vi "16 - Fonts (Render As Texture).vi"() -> ()   [LabVIEW 2015]
uses:
  Libraries/LibSDL2 Wrapper/Controls/Rectangle.ctl
  Libraries/LibSDL2 Wrapper/Controls/Init Flags.ctl
  Libraries/LibSDL2 Wrapper/Controls/NULL.ctl
  Libraries/LibSDL2 Wrapper/LibSDL2.lvlib
  Libraries/LibSDL2_Image Wrapper/LibSDL2_Image.lvlib
  Libraries/LibSDL2_TTF Wrapper/LibSDL2_TTF.lvlib
panel:
  out "Period":dbl format="%.2p"
  in  "milliseconds to wait":u32=250
  in  "Destination Rectangle":T1
  in  "Colour":u32(colorbox)=16448250
  in  "stop":bool
  out "Error":string
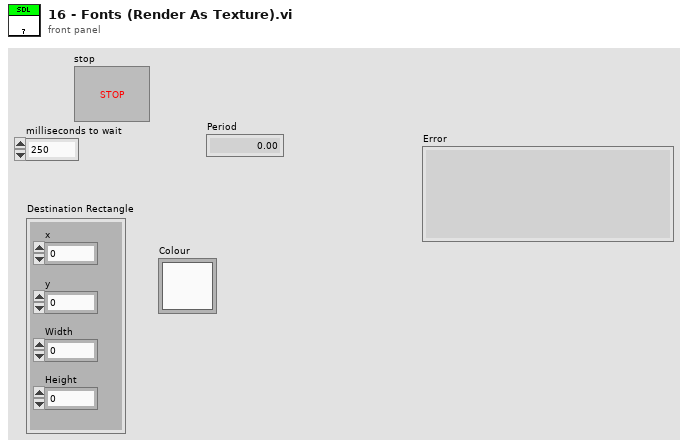
[diagram p1: front panel]
types:
  T1 = typedef "LibSDL2.lvlib/Rectangle.ctl" = cluster{"x":i32, "y":i32, "Width":i32, "Height":i32}
  T2 = typedef "LibSDL2.lvlib/Init Flags.ctl" = u32
  T3 = typedef "LibSDL2.lvlib/NULL.ctl" = enum32{"NULL"}
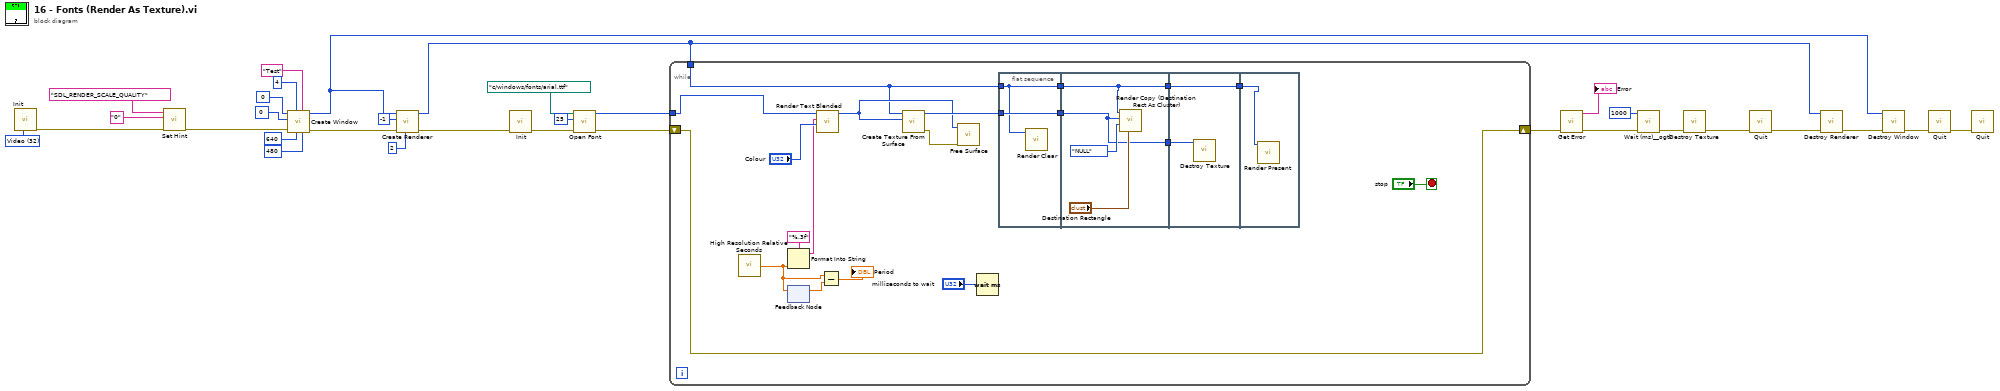
[diagram p0: block diagram]
diagram:
  w32 = T2 32 items=["Timer"=1, "Audio"=16, "Video"=32, "Joystick"=512, "Haptic"=4096, "Game Controller"=8192, "Events"=16384, "No Parachute"=1048576, "Everything"=17244689] ("Init Flags")
  n1 = call "Init.vi"("Flags"=w32) -> ("error out"=w23:errorcluster)  [unwired: 9 in, 1 out]
  n2 = call "Set Hint.vi"("error in"=w23, "Value"="0", "Name"="SDL_RENDER_SCALE_QUALITY") -> ("error out"=w22:errorcluster)  [unwired: 7 in, 1 out]
  n3 = call "Create Window.vi"("Height"=480, "Title"="Test", "Width"=640, "Flags"=u32 4, "error in"=w22, "Position y"=u32 0 ("Flags"), "Position x"=u32 0 ("Flags")) -> ("error out"=w2:errorcluster, "Window Pointer"=w7:u32)  [unwired: 3 in]
  n4 = call "Create Renderer.vi"("Flags"=u32 2, "error in"=w2, "Index"=-1, "Window Pointer"=w7) -> ("error out"=w1:errorcluster, "Renderer Pointer"=w3:u32)  [unwired: 6 in]
  n5 = call "Init.vi"("error in (no error)"=w1) -> ("error out"=w12:errorcluster)  [unwired: 9 in, 1 out]
  n6 = call "Open Font.vi"("error in (no error)"=w12, "Size"=25, "File"=path "c:/windows/fonts/arial.ttf") -> ("error out"=w11:errorcluster, "Font Pointer"=w10:u32)  [unwired: 7 in]
  n7 = while {
    tunnel: w10 -> [w48]
    shift-right: [w33] -> w6
    shift-left: w11 -> [w33]
    tunnel: w3 -> [w37]
    stop <- "stop" stop-if-true
    n8 = call <vilib>:"High Resolution Relative Seconds.vi"() -> ("relative seconds"=w41:dbl)
    n9 = Format Into String(format string="%.3f", w41) -> (resulting string=w45:string)  [unwired: 2 in, 1 out]
    n10 = feedback-in #1(w41) -> ()
    n11 = feedback #1() -> (w40:dbl)  [unwired: 1 in]
    n12 = call "Render Text Blended.vi"("Colour"="Colour", "Text"=w45, "Font Pointer"=w48) -> ("Surface Pointer"=w43:u32)  [unwired: 8 in]
    n13 = Subtract(x=w41, y=w40) -> (x-y=→"Period":dbl)
    n14 = call "Create Texture From Surface.vi"("Surface Pointer"=w43, "Renderer Pointer"=w37) -> ("error out"=w44:errorcluster, "Texture Pointer"=w47:u32)  [unwired: 8 in]
    n15 = call "Free Surface.vi"("error in"=w44, "Surface Pointer"=w43) -> ()  [unwired: 9 in, 1 out]
    n16 = Wait (ms)(milliseconds to wait="milliseconds to wait") -> ()  [unwired: 1 out]
    n17 = flat-sequence {
      tunnel: w47 -> [w53]
      tunnel: [w53] -> w38
      tunnel: w37 -> [w52]
      tunnel: [w52] -> w36
      tunnel: [w55] -> w42
      tunnel: w38 -> [w55]
      tunnel: w36 -> [w54]
      tunnel: [w54] -> w34
      tunnel: w42 -> [w59]
      tunnel: [w58] -> w35
      tunnel: w34 -> [w58]
      tunnel: w35 -> [w60]
      frame #0 {
        n18 = call "Render Clear.vi"("Renderer Pointer"=w52) -> ()  [unwired: 9 in, 2 out]
      }
      frame #1 {
        n19 = call "Render Copy (Destination Rect As Cluster).vi"("Destination Rectangle"="Destination Rectangle", "Source Rectangle Pointer"=NULL."NULL" ("Null"), "Texture Pointer"=w55, "Renderer Pointer"=w54) -> ()  [unwired: 7 in, 1 out]
      }
      frame #2 {
        n20 = call "Destroy Texture.vi"("Texture Pointer"=w59) -> ()  [unwired: 10 in, 1 out]
      }
      frame #3 {
        n21 = call "Render Present.vi"("Renderer Pointer"=w60) -> ()  [unwired: 10 in, 1 out]
      }
    }
  }
  n22 = call "Get Error.vi"("error in"=w6) -> ("error out"=w13:errorcluster, "Error"=→"Error":string)  [unwired: 9 in]
  n23 = call <userlib>:"Wait (ms)__ogtk.vi"("error in (no error)"=w13, "milliseconds to wait"=u32 1000) -> ("error out"=w14:errorcluster)  [unwired: 8 in, 1 out]
  n24 = call "Destroy Texture.vi"("error in"=w14) -> ("error out"=w17:errorcluster)  [unwired: 10 in]
  n25 = call "Quit.vi"("error in (no error)"=w17) -> ("error out"=w18:errorcluster)  [unwired: 10 in]
  n26 = call "Destroy Renderer.vi"("error in"=w18, "Renderer Pointer"=w3) -> ("error out"=w19:errorcluster)  [unwired: 9 in]
  n27 = call "Destroy Window.vi"("error in"=w19, "Window Pointer"=w7) -> ("error out"=w25:errorcluster)  [unwired: 9 in]
  n28 = call "Quit.vi"("error in"=w25) -> ("error out"=w24:errorcluster)  [unwired: 10 in]
  n29 = call "Quit.vi"("error in"=w24) -> ()  [unwired: 10 in, 1 out]
